vi "3_1.vi"() -> ()   [LabVIEW 2018]
panel:
  out "# de Iteraciones":dbl format="%#_4g"
  out "Curren number":dbl format="%#.2g"
  in  "number to match":dbl format="%#_4g"
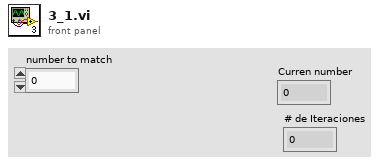
[diagram p1: front panel]
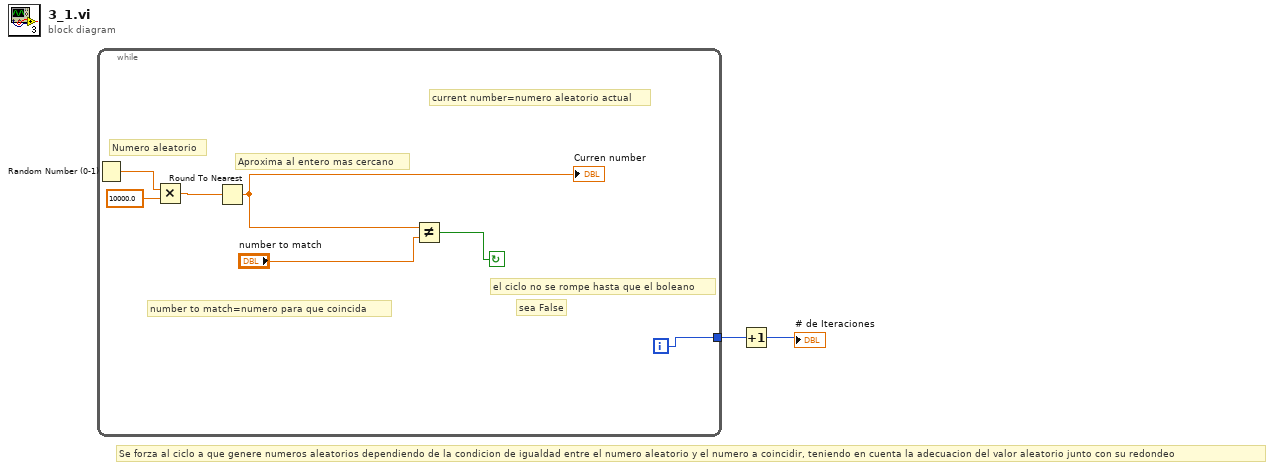
[diagram p0: block diagram]
diagram:
  # "Se forza al ciclo a que genere numeros aleatorios dependiendo de la condicion de igualdad entre el numero aleatorio y el numero a coincidir, teniendo en cuenta la adecuacion del valor aleatorio junto con su redondeo"
  n1 = while {
    tunnel: [w6] -> w2
    i -> [w6]
    stop <- w5 continue-if-true
    # "sea False"
    # "el ciclo no se rompe hasta que el boleano"
    # "Aproxima al entero mas cercano"
    # "Numero aleatorio"
    # "current number=numero aleatorio actual"
    # "number to match=numero para que coincida"
    n2 = Random Number (0-1)() -> (number: 0 to 1=w4:dbl)
    n3 = Multiply(x=w4, y=10000.0) -> (x*y=w3:dbl)
    n4 = Round To Nearest(number=w3) -> (nearest integer value=w8:dbl)
    "Curren number" <- w8
    n5 = Not Equal?(x=w8, y="number to match") -> (x != y?=w5:bool)
  }
  n6 = Increment(x=w2) -> (x+1=→"# de Iteraciones":i32)
